vi "APIrenovar token con refresh token 2020.vi"(9 "refresh_token":string, 10 "client_secret":string, 11 "client_id":string) -> (3 "access_token":string)   [LabVIEW 2025]
uses:
  <vilib>/httpClient/POSTBuffer.vi
  <vilib>/httpClient/LabVIEWHTTPClient.lvlib
panel:
  out "token_body":string
  out "token_response":string
  # "956292078384-6gohorktvdio30a79ptcb49shjdrcu5i.apps.googleusercontent.com"
  # "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"
  # "1//0f3gsYdYYOMD9CgYIARAAGA8SNwF-L9IrCeTTmbudkTk095Jv2oCWgXOoZcLXfY-3oiqVzWi7TTyNqoWFdHc_jsn3Wg0394NFuuE"
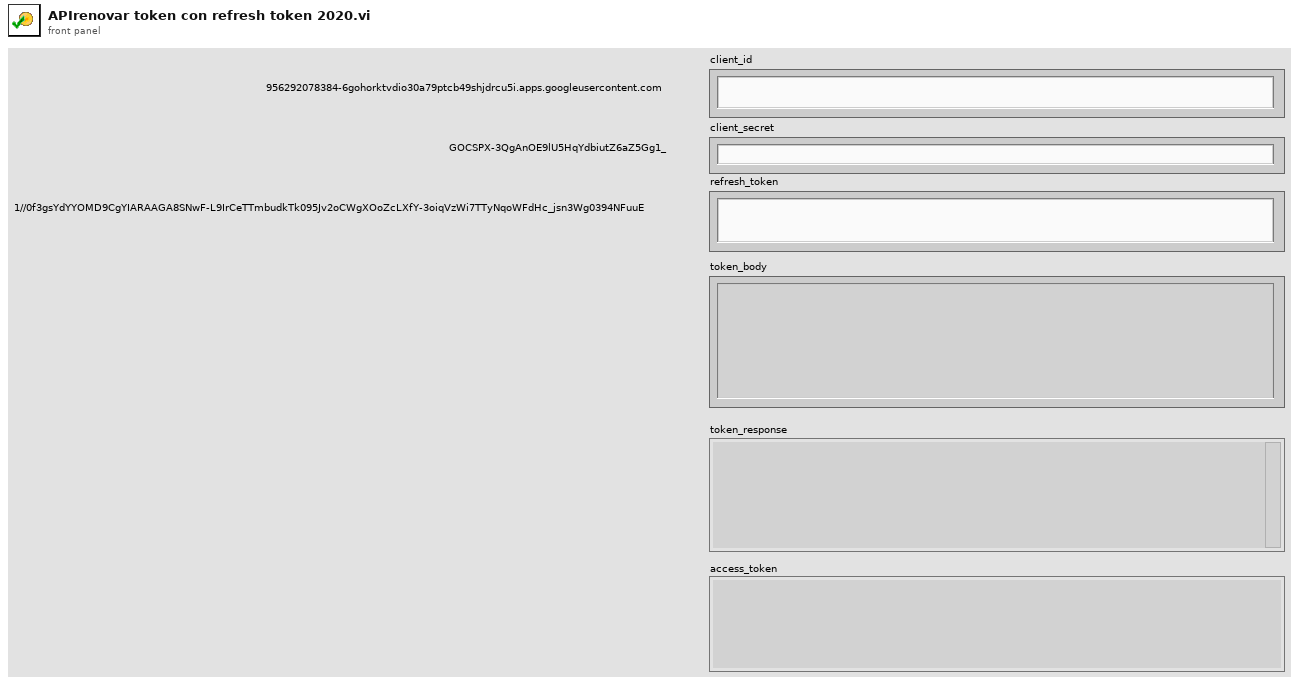
[diagram p1: front panel]
types:
  T1 = cluster{"access_token":string, "expires_in":i32, "scope":string, "token_type":string, "refresh_token_expires_in":i32}
  T2 = typedef "LabVIEWHTTPClient.lvlib/ClientHandle.ctl" = refnum<k1>
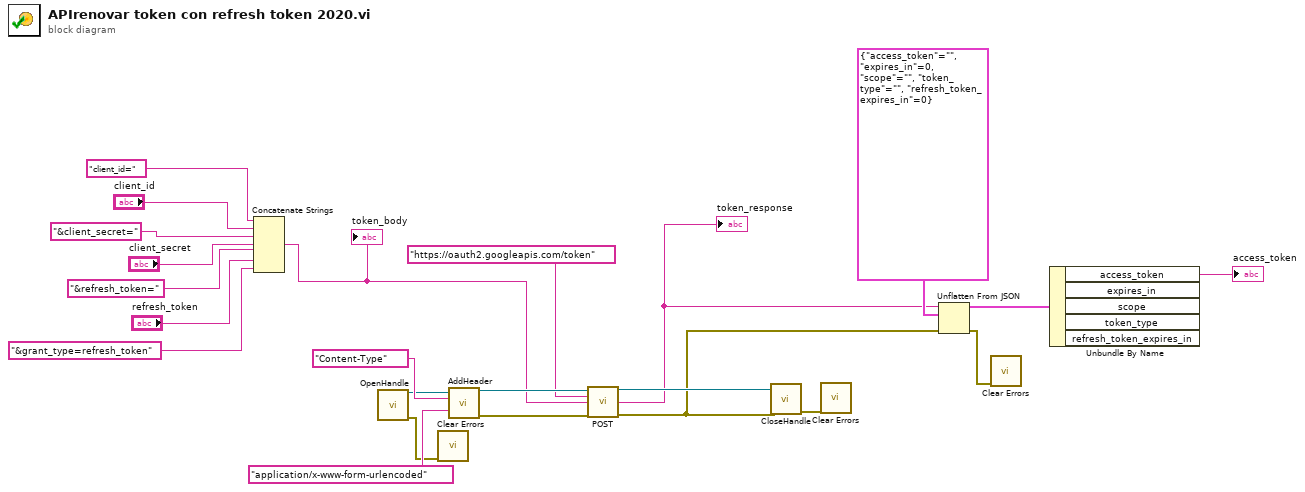
[diagram p0: block diagram]
diagram:
  n1 = Concatenate Strings("client_id=", "client_id", "&client_secret=", "client_secret", "&refresh_token=", "refresh_token", "&grant_type=refresh_token" ("redirect_uri")) -> (w5:string)
  "token_body" <- w5
  n2 = call <vilib>:"OpenHandle.vi"() -> ("client handle out"=w21:T2, "error out"=w1:errorcluster)  [unwired: 14 in]
  n3 = call <vilib>:"Clear Errors.vi"("error in (no error)"=w1) -> ()  [unwired: 5 in, 2 out]
  n4 = call <vilib>:"AddHeader.vi"("client handle"=w21, "header"="Content-Type", "value"="application/x-www-form-urlencoded") -> ("client handle out"=w20:T2, "error out"=w19:errorcluster)  [unwired: 11 in]
  n5 = call-poly <vilib>:"POST.vi"("client handle"=w20, "url"="https://oauth2.googleapis.com/token", "buffer"=w5, "error in (no error)"=w19) -> ("client handle out"=w18:T2, "body"=w7:string, "error out"=w4:errorcluster)  [unwired: 8 in, 1 out]
  "token_response" <- w7
  n6 = call <vilib>:"CloseHandle.vi"("client handle"=w18, "error in (no error)"=w4) -> ("error out"=w2:errorcluster)  [unwired: 13 in]
  n7 = call <vilib>:"Clear Errors.vi"("error in (no error)"=w2) -> ()  [unwired: 5 in, 2 out]
  n8 = Unflatten From JSON(JSON string=w7, type and defaults=T1 {"access_token"="", "expires_in"=0, "scope"="", "token_type"="", "refresh_token_expires_in"=0}, error in (no error)=w4) -> (value=w8:T1, error out=w3:errorcluster)  [unwired: 4 in]
  n9 = call <vilib>:"Clear Errors.vi"("error in (no error)"=w3) -> ()  [unwired: 5 in, 2 out]
  n10 = Unbundle By Name(w8) -> ("access_token"=→"access_token":string)  [unwired: 4 out]
